vi "Target Tracker.vi"() -> ()   [LabVIEW 2012]
uses:
  Robot Global Data.vi
  <vilib>/Rock Robotics/WPI/RobotDrive/WPI_RobotDriveGetSetRefNum.vi
  <vilib>/addons/control/pid/NI_PID_pid.lvlib
  <vilib>/addons/control/pid/pid.llb/PID (DBL).vi
panel:
  out "Enable Vision":bool
  in  "D":dbl
  in  "I":dbl
  in  "P":dbl
  out "Gauge":dbl(knob) scale=0.0..360.0
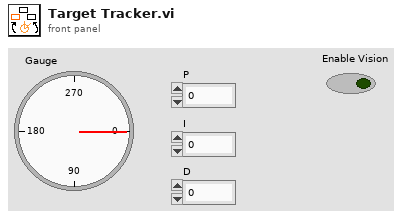
[diagram p1: front panel]
types:
  T1 = typedef "WPI_RobotDriveDevRef.ctl" = cluster{"DevStatus":errorcluster, "Motors[]":T2[], "Square Inputs":bool, "Max Output":dbl, "Isochronous":bool}
  T2 = typedef "WPI_MotorControlDeviceRef.ctl" = cluster{"DeviceStatus":errorcluster, "Type":enum16{"PWM", "CAN"}, "PWM":cluster{"Digital Module":T3, "PWM Channel":T4, "DeadBand":T5}, "CAN":cluster{"Device Number":u8, "Control Mode":T6, "Semaphore":T7, "Max Vout":dbl}, "Invert":bool, "TransformRef":T8, "InvTransformRef":T8}
  T3 = typedef "FPGA_TypedefDigitalModule.ctl" = enum16{"Digital Module 1", "Digital Module 2"}
  T4 = typedef "FPGA_DIOPWMChannel.ctl" = enum8{"PWM 1", "PWM 2", "PWM 3", "PWM 4", "PWM 5", "PWM 6", "PWM 7", "PWM 8", "PWM 9", "PWM 10", "Invalid"}
  T5 = typedef "WPI_PWMDeadband.ctl" = cluster{"Name":string, "maxPositivePwm":i32, "minPositivePwm":i32, "centerPwm":i32, "maxNegativePwm":i32, "minNegativePwm":i32, "angularRange":u16}
  T6 = typedef "WPI_CANJaguar_ControlMode.ctl" = enum8{"Percent VBus", "Current", "Speed", "Position", "Voltage"}
  T7 = typedef "Semaphore RefNum" = refnum<k1>
  T8 = typedef "WPI_PWMTransform_ConPane.ctl" = refnum<vi>
  T9 = typedef "WPI_GyroDevRef.ctl" = cluster{"DevStatus":errorcluster, "Analog Module":T10, "Analog Channel":T11, "Offset":dbl, "Gain (VoltsPerDegree/Second)":dbl}
  T10 = typedef "FPGA_TypedefAnalogModule.ctl" = enum16{"Analog Module 1", "Analog Module 2"}
  T11 = typedef "FPGA_AIChannel.ctl" = enum8{"AI 1", "AI 2", "AI 3", "AI 4", "AI 5", "AI 6", "AI 7", "AI 8", "Invalid"}
  T12 = cluster{"proportional gain (Kc)":dbl, "integral time (Ti, min)":dbl, "derivative time (Td, min)":dbl}
  T13 = cluster{"Position":cluster{"X":dbl, "Y":dbl}, "Distance (ft)":dbl}[]
  T14 = cluster{"Position":cluster{"X":dbl, "Y":dbl}, "Distance (ft)":dbl}
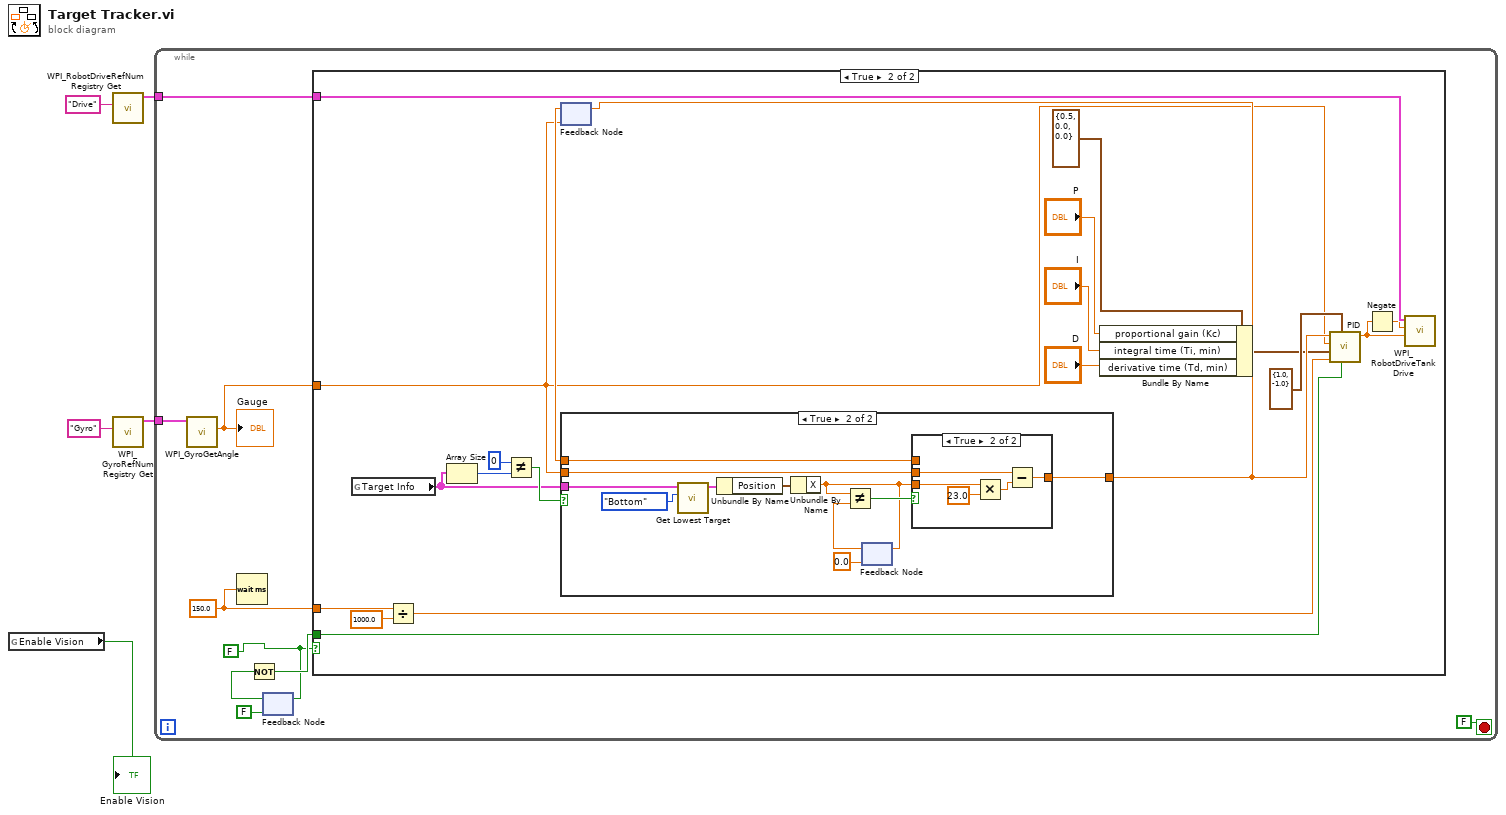
[diagram p0: block diagram]
diagram:
  n1 = global read "Robot Global Data.vi" "Enable Vision"() -> (→"Enable Vision":bool)
  n2 = call <vilib>:"WPI_RobotDriveRefNum Registry Get.vi"("refnum name"="Drive") -> ("RobotDriveDevRef"=w2:T1)  [unwired: 9 in, 1 out]
  n3 = call <vilib>:"WPI_GyroRefNum Registry Get.vi"("refnum name"="Gyro") -> ("GyroDevRef"=w3:T9)  [unwired: 9 in, 1 out]
  n4 = while {
    tunnel: w3 -> [w8]
    tunnel: w2 -> [w10]
    stop <- FALSE stop-if-true
    w6 = FALSE
    w9 = 150.0
    n5 = call <vilib>:"WPI_GyroGetAngle.vi"("GyroDevRef"=w8) -> ("Angle"=w7:dbl)  [unwired: 7 in, 3 out]
    "Gauge" <- w7
    n6 = Wait (ms)(milliseconds to wait=w9) -> ()  [unwired: 1 out]
    n7 = feedback-in #1(w6) -> ()
    n8 = feedback #1(FALSE) -> (w12:bool)
    n9 = Not(x=w12) -> (.not. x?=w11:bool)
    n10 = case shown="True" w6 {
      tunnel: w11 -> [_ w33]
      tunnel: w9 -> [_ w23]
      tunnel: w10 -> [_ w27]
      tunnel: w7 -> [_ w20]
      frame False {
      }
      frame True {
        n11 = global read "Robot Global Data.vi" "Target Info"() -> (w28:T13)
        n12 = Divide(x=w23, y=1000.0) -> (x/y=w21:dbl)
        n13 = Array Size(array=w28) -> (size(s)=w30:i32)
        n14 = Not Equal?(x=0, y=w30) -> (x != y?=w31:bool)
        n15 = feedback #2(w20) -> (w32:dbl)
        n16 = case shown="True" w31 {
          tunnel: w32 -> [w35 w37]
          tunnel: w28 -> [_ w46]
          tunnel: w20 -> [_ w39]
          tunnel: [w35 w38] -> w24
          frame False {
          }
          frame True {
            n17 = call "Get Lowest Target.vi"("Enum"=enum16{"Top", "Right", "Bottom", "Left"}."Bottom", "Target Info"=w46) -> ("Cluster"=w45:T14)  [unwired: 9 in]
            n18 = Unbundle By Name(w45) -> ("Position"=w44:cluster{"X":dbl, "Y":dbl})
            n19 = Unbundle By Name(w44) -> ("X"=w40:dbl)
            n20 = feedback-in #3(w40) -> ()
            n21 = feedback #3(0.0) -> (w41:dbl)
            n22 = Not Equal?(x=w40, y=w41) -> (x != y?=w42:bool)
            n23 = case shown="True" w42 {
              tunnel: w40 -> [_ w51]
              tunnel: w39 -> [_ w49]
              tunnel: [w47 w48] -> w38
              tunnel: w37 -> [w47 _]
              frame False {
              }
              frame True {
                n24 = Multiply(x=w51, y=23.0) -> (x*y=w50:dbl)
                n25 = Subtract(x=w49, y=w50) -> (x-y=w48:dbl)
              }
            }
          }
        }
        n26 = feedback-in #2(w24) -> ()
        n27 = Bundle By Name(cluster=T12 {"proportional gain (Kc)"=0.5, "integral time (Ti, min)"=0.0, "derivative time (Td, min)"=0.0} ("PID gains"), "proportional gain (Kc)"="P", "integral time (Ti, min)"="I", "derivative time (Td, min)"="D") -> (w15:T12)
        n28 = call-poly <vilib>:"PID.vi"("reinitialize? (F)"=w33, "output range"=cluster{"output high":dbl, "output low":dbl} {"output high"=1.0, "output low"=-1.0}, "dt (s)"=w21, "PID gains"=w15, "process variable"=w20, "setpoint"=w24) -> ("output"=w26:dbl)  [unwired: 4 in, 1 out]
        n29 = Negate(x=w26) -> (-x=w25:dbl)
        n30 = call <vilib>:"WPI_RobotDriveTankDrive.vi"("Right axis value"=w26, "Left axis value"=w25, "RobotDriveDevRef"=w27) -> ()  [unwired: 6 in, 3 out]
      }
    }
  }
